vi "Configure Output Impedance.vi"(8 "error in (no error)":errorcluster, 9 "Output Impedance (50 Ohm)":i32=50, 10 "Output Channel (1: Channel 1)":i32(ring)=1 items=["Channel 1"=1, "Channel 2"=2], 11 "VISA resource name":refnum<visa-resource-name>) -> (0 "error out":errorcluster, 3 "VISA resource name out":refnum<visa-resource-name>)   [LabVIEW 2015, in "RIGOL DG4000 Series.lvlib"]
doc: "Configures the output impedance for the function generator."
uses:
  <instrlib>/RIGOL DG4000 Series/RIGOL DG4000 Series.lvlib
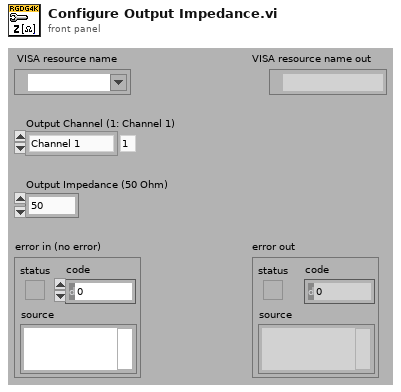
[diagram p1: front panel]
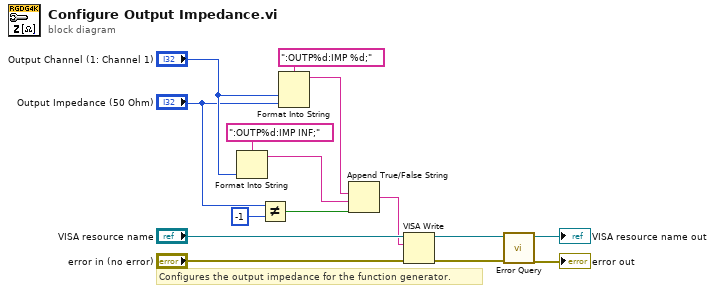
[diagram p0: block diagram]
diagram:
  # "Configures the output impedance for the function generator."
  n1 = Format Into String(format string=":OUTP%d:IMP INF;", "Output Channel (1: Channel 1)") -> (resulting string=w2:string)  [unwired: 2 in, 1 out]
  n2 = Not Equal?(x="Output Impedance (50 Ohm)", y=-1) -> (x != y?=w3:bool)
  n3 = Format Into String(format string=":OUTP%d:IMP %d;", "Output Channel (1: Channel 1)", "Output Impedance (50 Ohm)") -> (resulting string=w6:string)  [unwired: 2 in, 1 out]
  n4 = Append True/False String(1:w3, 2:w2, 3:w6) -> (0:w1:string)  [unwired: 1 out]
  n5 = VISA Write(VISA resource name="VISA resource name", write buffer=w1, error in (no error)="error in (no error)") -> (VISA resource name out=w12:refnum<visa-resource-name>, error out=w11:errorcluster)  [unwired: 1 out]
  n6 = call <instrlib>:"Error Query.vi"("error in (no error)"=w11, "VISA resource name"=w12) -> ("error out"=→"error out":errorcluster, "VISA resource name out"=→"VISA resource name out":refnum<visa-resource-name>)  [unwired: 8 out]
